vi "Scpi_test2.vi"() -> ()   [LabVIEW 2009]
panel:
  in  "Command":string
  out "error out 2":errorcluster
  in  "Instrument":T1(ring)
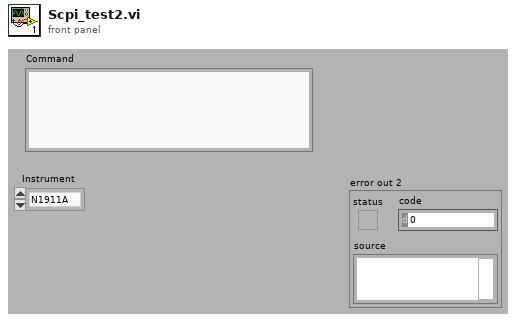
[diagram p1: front panel]
types:
  T1 = enum16{"N1911A", "Siggen", "34980a", "E4418B", "Rvp8"}
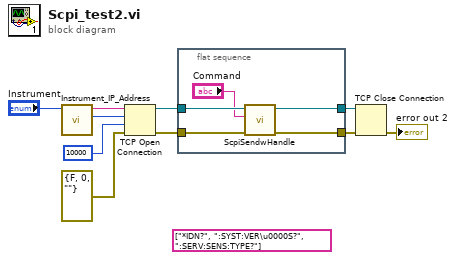
[diagram p0: block diagram]
diagram:
  (unwired) string[] ["*IDN?", ":SYST:VER\u0000S?", ":SERV:SENS:TYPE?"] ("Array")
  n1 = call "Instrument_IP_Address.vi"("Instrument"="Instrument") -> ("Port"=w8:u16, "IP Address"=w9:string)  [unwired: 9 in]
  n2 = TCP Open Connection(address=w9, remote port or service name=w8, timeout ms (60000)=10000, error in (no error)=errorcluster {"status"=FALSE, "code"=0, "source"=""}) -> (connection ID=w4:refnum<k5>, error out=w5:errorcluster)  [unwired: 1 in]
  n3 = flat-sequence {
    tunnel: w5 -> [w14]
    tunnel: [w13] -> w2
    tunnel: [w12] -> w3
    tunnel: w4 -> [w15]
    frame #0 {
      n4 = call "ScpiSendwHandle.vi"("error in (no error)"=w14, "Command"="Command", "connection ID"=w15) -> ("error out"=w13:errorcluster, "connection ID out"=w12:refnum<k5>)  [unwired: 7 in]
    }
  }
  n5 = TCP Close Connection(connection ID=w3, error in (no error)=w2) -> (error out=→"error out 2":errorcluster)  [unwired: 1 in, 1 out]
